vi "Error Handler - Confirm Quit.vi"() -> (2 "exit confirmed":bool=TRUE, 3 "channel":T1)   [LabVIEW 2019]
doc: "Queries the user to find out if the application should exit or not."
uses:
  03.3 Queued Message Handler/support/Message Queue/Message Queue.lvlib
  Producer Consumer (Events)/support/Message Queue/Message Cluster.ctl
  <extravilib>/ChannelInstances/Messenger-t'Message Queue.lvlib-Message Cluster.ctl'/))Channel.ctl
  <extravilib>/ChannelInstances/Messenger-t'Message Queue.lvlib-Message Cluster.ctl'.lvlib
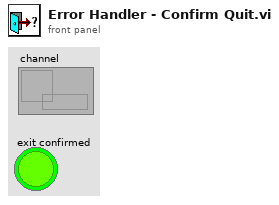
[diagram p1: front panel]
types:
  T1 = typedef "Messenger-t'Message Queue.lvlib-Message Cluster.ctl'.lvlib/))Channel.ctl" = refnum<queue>
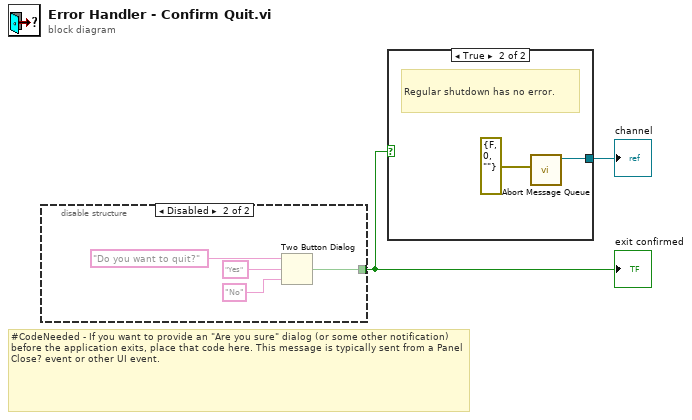
[diagram p0: block diagram]
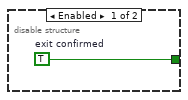
[diagram p3: hidden frame]
diagram:
  # "#CodeNeeded - If you want to provide an \"Are you sure\" dialog (or some other notification) before the application exits, place that code here. This message is typically sent from a Panel Close? event or other UI event."
  n1 = disable-structure shown="Disabled" {
    disable-tunnel: [w3 w4] -> w1
    frame Enabled {
      w3 = TRUE  # exit confirmed
    }
    frame Disabled {
      n2 = Two Button Dialog(message="Do you want to quit?" ("Do you want to quit?"), 1:"No" ("No"), 2:"Yes" ("Yes")) -> (T button?=w4:bool)
    }
  }
  "exit confirmed" <- w1
  n3 = case shown="True" w1 {
    tunnel: [_ w9] -> w2
    frame False {
    }
    frame True {
      # "Regular shutdown has no error."
      n4 = call "Abort Message Queue.vi"("error to report"=errorcluster {"status"=FALSE, "code"=0, "source"=""} ("error IO")) -> ("channel"=w9:T1)  [unwired: 10 in]
    }
  }
  "channel" <- w2
